vi "WPI_CameraSet Sharpness.vi"(8 "error in (no error)":errorcluster, 10 "Sharpness":i32 min=0 max=100, 11 "CameraDevRef":T1={"Camera Address"="192.168.0.90", "CameraStatus"={"status"=FALSE, "code"=0, "source"=""}}) -> (0 "error out":errorcluster, 3 "CameraDevRef Out":T1)   [LabVIEW 2017]
doc: "Specifies the sharpness setting of the camera you specify.\n\nThis software is licensed. Open the labview\\readme\\WPI Robotics Library Open Source License.txt file for more information."
uses:
  <vilib>/Rock Robotics/WPI/Camera/WPI_CameraDevRef.ctl
  <vilib>/Rock Robotics/WPI/Camera/WPI_CameraSettings Operations.ctl
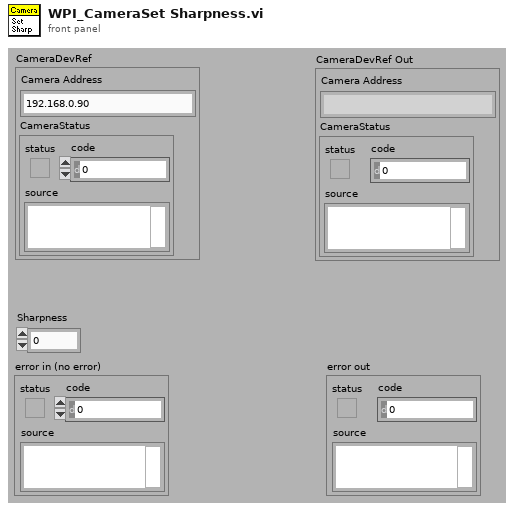
[diagram p1: front panel]
types:
  T1 = typedef "WPI_CameraDevRef.ctl" = cluster{"Camera Address":string, "CameraStatus":errorcluster}
  T2 = typedef "WPI_CameraSettings Operations.ctl" = enum16{"Udate FPS", "Update Compression", "Update Size", "Update White Balance", "Update Brightness", "Update Sharpness", "Update Exposure", "Update Exposure Value", "Update Color Level", "Update Exp Priority", "Update Color Enable", "Update JPG", "Update MJPG", "Read and Clear", "Read", "Init"}
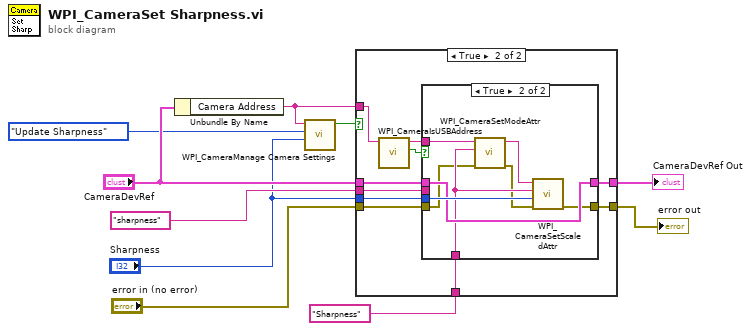
[diagram p0: block diagram]
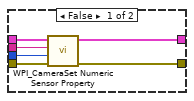
[diagram p3: hidden frame]
diagram:
  n1 = Unbundle By Name("CameraDevRef") -> ("Camera Address"=w2:string)
  n2 = call <vilib>:"WPI_CameraManage Camera Settings.vi"("Value"="Sharpness", "Operation"=WPI_CameraSettings_Operations."Update Sharpness", "Camera IP"=w2) -> ("Changed"=w5:bool)  [unwired: 7 in, 1 out]
  n3 = case shown="True" w5 {
    tunnel: "CameraDevRef" -> [w12 w22]
    tunnel: "sharpness" ("Property Name") -> [_ w21]
    tunnel: "Sharpness" -> [_ w20]
    tunnel: [w12 w19] -> w9
    tunnel: "error in (no error)" -> [w11 w18]
    tunnel: [w11 w17] -> w7
    tunnel: w2 -> [_ w14]
    tunnel: "Sharpness" -> [_ w13]
    frame False {
    }
    frame True {
      n4 = call <vilib>:"WPI_CameraIsUSBAddress.vi"("Camera Address In"=w14) -> ("USB?"=w16:bool, "Camera Address Out"=w15:string)  [unwired: 8 in, 1 out]
      n5 = case shown="True" w16 {
        tunnel: w22 -> [w28 w34]
        tunnel: w21 -> [w27 _]
        tunnel: w20 -> [w26 w36]
        tunnel: [w25 w34] -> w19
        tunnel: w18 -> [w24 w31]
        tunnel: [w23 w29] -> w17
        tunnel: w15 -> [_ w33]
        tunnel: w13 -> [_ w32]
        frame False {
          n6 = call <vilib>:"WPI_CameraSet Numeric Sensor Property.vi"("error in (no error)"=w24, "Value"=w26, "Property Name"=w27, "CameraDevRef"=w28) -> ("error out"=w23:errorcluster, "CameraDevRef out"=w25:T1)  [unwired: 4 in, 2 out]
        }
        frame True {
          n7 = call <vilib>:"WPI_CameraSetModeAttr.vi"("error in (no error)"=w31, "Attr String"=w32, "Camera Address In"=w33) -> ("error out"=w30:errorcluster, "Camera Address Out"=w35:string)  [unwired: 7 in]
          n8 = call <vilib>:"WPI_CameraSetScaledAttr.vi"("error in (no error)"=w30, "Scaled"=w36, "Attr String"=w32, "Camera Address In"=w35) -> ("error out"=w29:errorcluster)  [unwired: 6 in, 1 out]
        }
      }
    }
  }
  "CameraDevRef Out" <- w9
  "error out" <- w7
